vi "Send-Trigger.vi"(8 "error in (no error)":errorcluster, 10 "Trigger mode":T1=enum."Framegrabber timed (sync.)", 11 "PF_MV1-D1312-240 in":refnum<class "PF_MV1-D1312-240.lvclass">) -> (0 "error out":errorcluster, 3 "PF_MV1-D1312-240 out":refnum<class "PF_MV1-D1312-240.lvclass">)   [LabVIEW 2013, in "CameraVision.lvlib" / "PF_MV1-D1312-240.lvclass"]
uses:
  PF_MV1-D1312-240.lvclass
  Main/Acquisition/Trigger-modes.ctl
  Camera.lvclass/Camera.ctl
  Camera.lvclass
  <userlib>/Photonfocus Toolkit/Photonfocus_Toolkit.lvlib
  Main/Acquisition/CV-Acquisition.lvclass
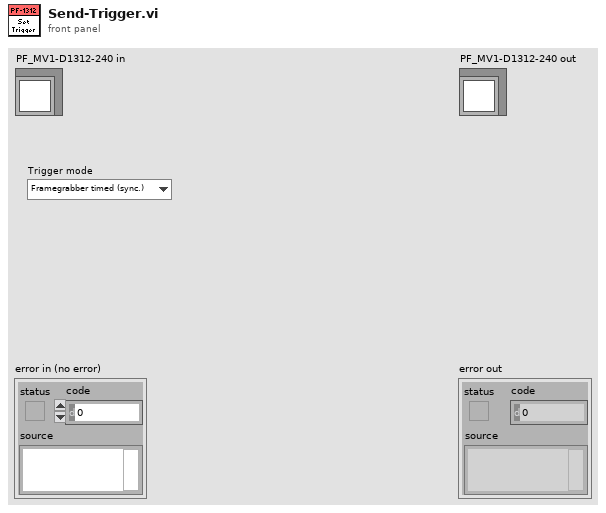
[diagram p1: front panel]
types:
  T1 = typedef "CameraVision.lvlib/CV-Acquisition.lvclass/Trigger-modes.ctl" = enum16{"Camera timed (not sync.)", "Framegrabber timed (sync.)", "Software timed (sync.)", "External timing (sync.)", "Manual (sync.)", "Gated - camera (not sync.)", "Gated - grabber (sync.)", "Gated - software (sync.)", "Gated - external (sync.)"}
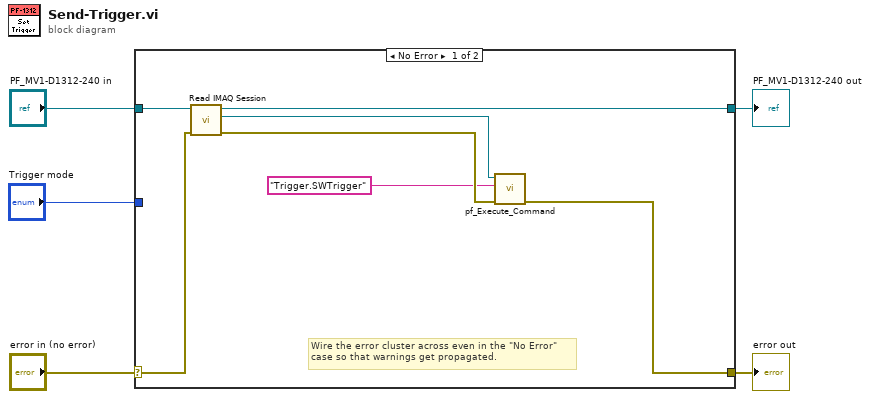
[diagram p0: block diagram]
diagram:
  n1 = case shown="No Error" "error in (no error)" {
    selector: "error in (no error)" -> [w10 w14]
    tunnel: [w9 w14] -> w4
    tunnel: [w11 w13] -> w2
    tunnel: "PF_MV1-D1312-240 in" -> [w12 w13]
    tunnel: "Trigger mode" -> [_ _]
    frame No Error {
      # "Wire the error cluster across even in the \"No Error\"\ncase so that warnings get propagated."
      n2 = call "Read IMAQ Session.vi"("error in (no error)"=w10, "Camera in"=w12) -> ("error out"=w8:errorcluster, "IMAQ Session"=w7:refnum<k11>, "Camera out"=w11:refnum<class "PF_MV1-D1312-240.lvclass">)  [unwired: 7 in]
      n3 = call <userlib>:"pf_Execute_Command.vi"("error in (no error)"=w8, "Command"="Trigger.SWTrigger" ("Property Name"), "IMAQ Session in"=w7) -> ("error out"=w9:errorcluster)  [unwired: 7 in, 1 out]
    }
    frame Error {
    }
  }
  "error out" <- w4
  "PF_MV1-D1312-240 out" <- w2
